vi "start.vi"(8 "error in (no error)":errorcluster, 9 "command_start_Ctl out":T1, 10 "commandID":i32, 11 "CommandConstruction in":refnum<class "CommandConstruction.lvclass">) -> (0 "error out":errorcluster, 3 "CommandConstruction out":refnum<class "CommandConstruction.lvclass">)   [LabVIEW 2016, in "CommandConstruction.lvclass"]
uses:
  CommandConstruction.lvclass
  ICommandFactory/ICommandFactory.lvclass
  Commands/Start/Start.lvclass
  Typedefs/CommandValue.ctl
  home/andres/ct_cmpuserevents/CommandThisComponent/CommandThisComponent.lvclass
  home/andres/ct_cmpuserevents/ComponentTemplateCore/ComponentModel/ComponentModel/Command/Command.lvclass
  ts_sallv_exa/DataTypes/command_start.ctl
  Desktop/TestConnectRelease/SALLV_EXA.lvlib
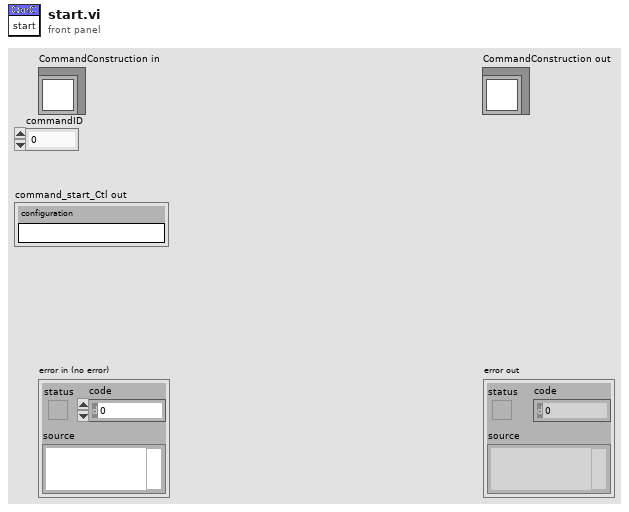
[diagram p1: front panel]
types:
  T1 = typedef "SALLV_EXA.lvlib/command_start.ctl" = cluster{"configuration":string}
  T2 = typedef "CommandValue.ctl" = enum16{"ClearError", "Disable", "Enable", "Exit", "GoToStandby", "OnHeartbeat", "OnIncomingMessagingError", "OnInterrupt", "Start"}
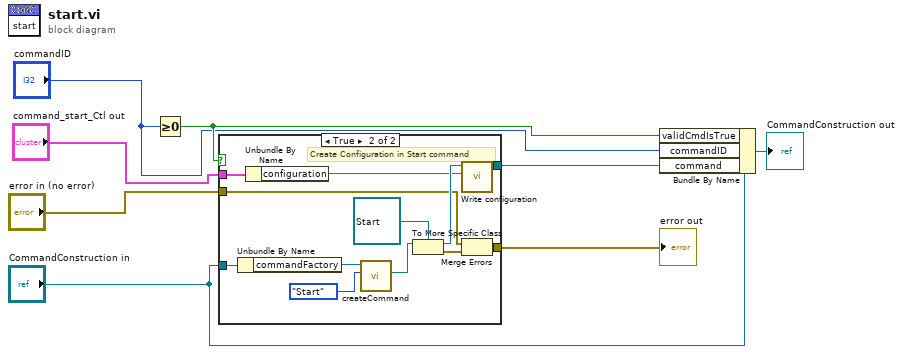
[diagram p0: block diagram]
diagram:
  n1 = Greater Or Equal To 0?(x="commandID") -> (x >= 0?=w6:bool)
  n2 = case shown="True" w6 {
    tunnel: [w9 w13] -> w8
    tunnel: "error in (no error)" -> [w9 w11]
    tunnel: "CommandConstruction in" -> [_ w20]
    tunnel: "command_start_Ctl out" -> [_ w19]
    tunnel: [_ w12] -> w5
    frame False {
    }
    frame True {
      # "Create Configuration in Start command"
      n3 = Unbundle By Name(w20) -> ("commandFactory"=w21:refnum<class "ICommandFactory.lvclass">)
      n4 = Unbundle By Name(w19) -> ("configuration"=w15:string)
      n5 = call-dynamic "createCommand.vi"("commandValue"=CommandValue."Start", "ICommandFactory in"=w21) -> ("command"=w17:refnum<class "Command.lvclass">)  [unwired: 7 in, 2 out]
      n6 = To More Specific Class(target class=refnum<class "Start.lvclass"> refnum ("Commands.lvlib:Start.lvclass"), reference=w17) -> (specific class reference=w16:refnum<class "Start.lvclass">, error out=w14:errorcluster)  [unwired: 1 in]
      n7 = call "Write configuration.vi"("configuration"=w15, "Start in"=w16) -> ("Start out"=w12:refnum<class "Start.lvclass">)  [unwired: 9 in]
      n8 = Merge Errors(w11, w14) -> (w13:errorcluster)
    }
  }
  "error out" <- w8
  n9 = Bundle By Name(cluster="CommandConstruction in", "validCmdIsTrue"=w6, "commandID"="commandID", "command"=w5) -> (→"CommandConstruction out":refnum<class "CommandConstruction.lvclass">)
